vi "Zadanie 1.vi"() -> ()   [LabVIEW 2020]
panel:
  out "BUFFER 2":bool
  in  "Przycisk BUFFER 2":bool
  out "NAND":bool
  in  "Pzycisk NAND 2":bool
  in  "Przycisk NAND 1":bool
  out "NOR":bool
  in  "Przycisk NOR 2":bool
  in  "Przycisk NOR 1":bool
  out "OR":bool
  in  "Przycisk OR 2":bool
  in  "Przycisk OR 1":bool
  in  "Przycisk AND 2":bool
  out "AND":bool
  in  "Przycisk AND 1":bool
  out "BUFFER":bool
  in  "Przycisk BUFFER":bool
  in  "Halt baby":bool
  out "NOT":bool
  in  "Przycisk NOT":bool
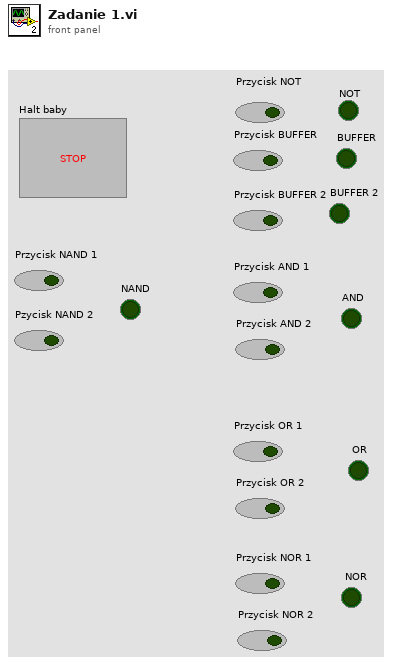
[diagram p1: front panel]
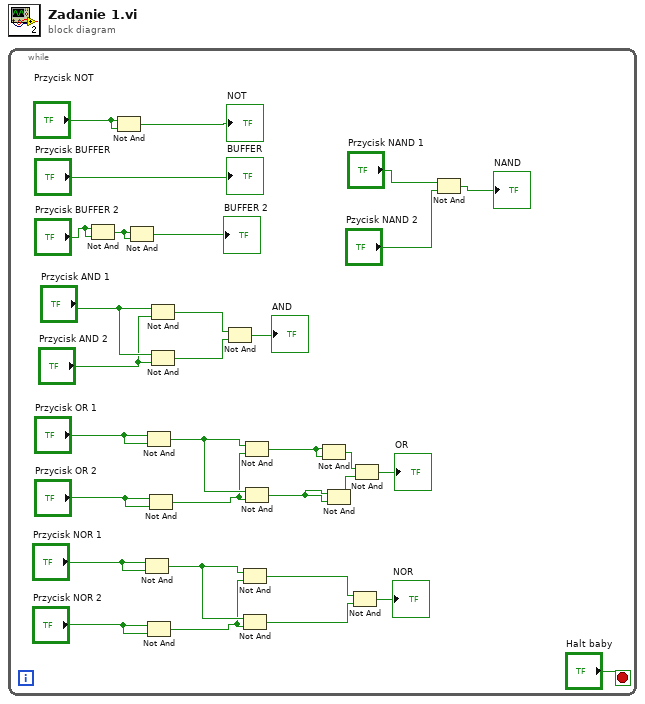
[diagram p0: block diagram]
diagram:
  n1 = while {
    stop <- "Halt baby" stop-if-true
    n2 = Not And(1:"Przycisk BUFFER 2", 2:"Przycisk BUFFER 2") -> (0:w2:bool)
    n3 = Not And(1:"Przycisk NOT", 2:"Przycisk NOT") -> (0:→"NOT":bool)
    n4 = Not And(1:w2, 2:w2) -> (0:→"BUFFER 2":bool)
    n5 = Not And(1:"Przycisk NOR 1", 2:"Przycisk NOR 1") -> (0:w11:bool)
    n6 = Not And(1:"Przycisk OR 1", 2:"Przycisk OR 1") -> (0:w20:bool)
    n7 = Not And(1:"Przycisk NOR 2", 2:"Przycisk NOR 2") -> (0:w10:bool)
    n8 = Not And(1:"Przycisk OR 2", 2:"Przycisk OR 2") -> (0:w19:bool)
    n9 = Not And(1:"Przycisk AND 2", 2:"Przycisk AND 1") -> (0:w25:bool)
    n10 = Not And(1:"Przycisk AND 2", 2:"Przycisk AND 1") -> (0:w24:bool)
    n11 = Not And(1:w24, 2:w25) -> (0:→"AND":bool)
    n12 = Not And(1:w10, 2:w11) -> (0:w8:bool)
    n13 = Not And(1:w10, 2:w11) -> (0:w7:bool)
    n14 = Not And(1:w19, 2:w20) -> (0:w18:bool)
    n15 = Not And(1:w19, 2:w20) -> (0:w17:bool)
    n16 = Not And(1:w18, 2:w18) -> (0:w16:bool)
    n17 = Not And(1:w17, 2:w17) -> (0:w15:bool)
    n18 = Not And(1:w7, 2:w8) -> (0:→"NOR":bool)
    n19 = Not And(1:w15, 2:w16) -> (0:→"OR":bool)
    n20 = Not And(1:"Pzycisk NAND 2", 2:"Przycisk NAND 1") -> (0:→"NAND":bool)
    "BUFFER" <- "Przycisk BUFFER"
  }
